vi "Request For Image.vi"(8 "error in (no error)":errorcluster, 9 "Caller Messge":refnum<class "Image Msg.lvclass">, 10 "Caller Enqueuer":refnum<class "Message Enqueuer.lvclass">, 11 "Image Acquisition in":refnum<class "Image Acquisition.lvclass">) -> (0 "error out":errorcluster, 3 "Image Acquisition out":refnum<class "Image Acquisition.lvclass">)   [LabVIEW 2016, in "Image Acquisition.lvlib" / "Image Acquisition.lvclass"]
uses:
  Image Acquisition.lvclass
  <vilib>/ActorFramework/Message Enqueuer/Message Enqueuer.lvclass
  Image Acquisition Messages/Image Msg/Image Msg.lvclass
  C:/Program Files (x86)/National Instruments/LabVIEW 2016/vi.lib/ActorFramework/Message/Message.lvclass
  Image Acquisition.lvclass/Image Acquisition.ctl
  Image Acquisition Messages/Image Msg/Image Msg.lvclass/Image Msg.ctl
  <vilib>/ActorFramework/Message Enqueuer/Message Enqueuer.lvclass/Message Enqueuer.ctl
  <vilib>/ActorFramework/Message Enqueuer/Enqueue.vi
  <vilib>/ActorFramework/Message Priority Queue/Priority Enqueue.vi
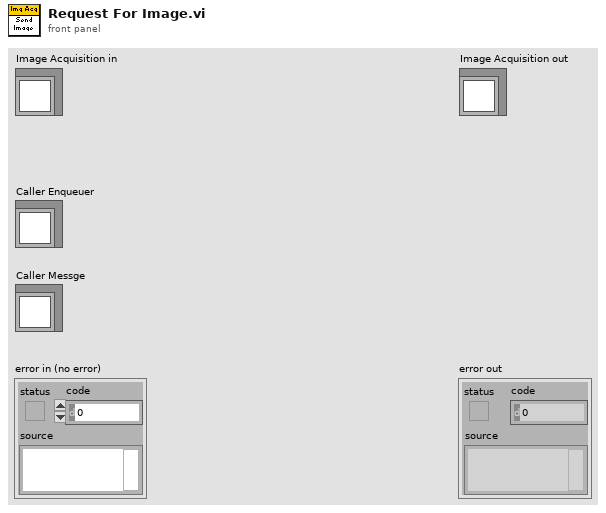
[diagram p1: front panel]
types:
  T1 = typedef "IMAQ Image.ctl" = refnum<image>
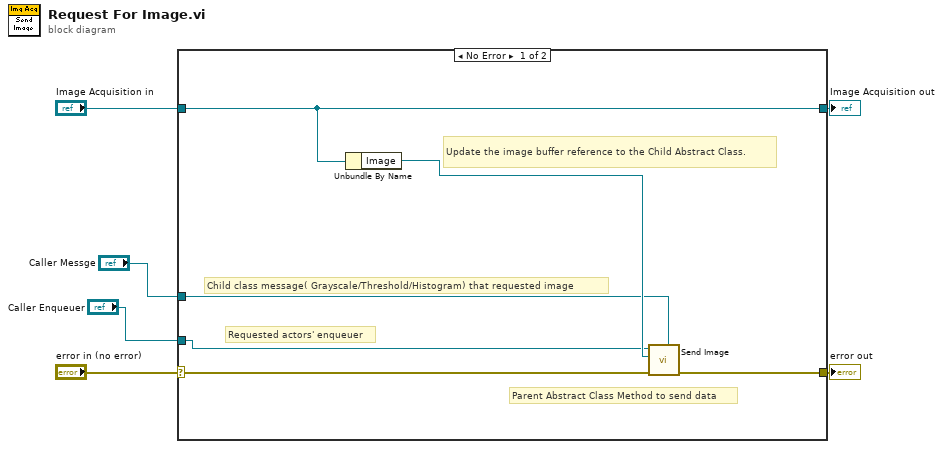
[diagram p0: block diagram]
diagram:
  n1 = case shown="No Error" "error in (no error)" {
    selector: "error in (no error)" -> [w8 w14]
    tunnel: [w7 w14] -> w5
    tunnel: [w12 w13] -> w3
    tunnel: "Image Acquisition in" -> [w12 w13]
    tunnel: "Caller Messge" -> [w9 _]
    tunnel: "Caller Enqueuer" -> [w10 _]
    frame No Error {
      # "Requested actors' enqueuer"
      # "Child class message( Grayscale/Threshold/Histogram) that requested image"
      # "Parent Abstract Class Method to send data"
      # "Update the image buffer reference to the Child Abstract Class."
      n2 = Unbundle By Name(w12) -> ("Image"=w11:T1)
      n3 = call "Send Image.vi"("Message Type"=w9, "error in (no error)"=w8, "Image"=w11, "Message Enqueuer"=w10) -> ("error out"=w7:errorcluster)  [unwired: 6 in, 1 out]
    }
    frame Error {
    }
  }
  "error out" <- w5
  "Image Acquisition out" <- w3
